vi "Workspace.UI.Update.vi"(8 "error in (no error)":errorcluster, 9 "Data.PendingChange?":bool, 10 "Values":dbl[](array[numeric]), 11 "UI.Refs":T1) -> (0 "error out":errorcluster)   [LabVIEW 2019, in "Diagnostics Workspace Shared.lvlib"]
uses:
  Diagnostics Workspace Shared.lvlib
  Types/UI.Refs.ctl
  Addon/Addon Shared/Types/Command.New.ctl
  SubModules/CAN-Streaming-Support/Source/Addon/Addon Shared/Types/Type Filter.ctl
  Addon/Addon Shared/Diagnostics Addon Shared.lvlib
  SubModules/CAN-Streaming-Support/Source/Addon/Addon Shared/CAN Stream Support Shared.lvlib
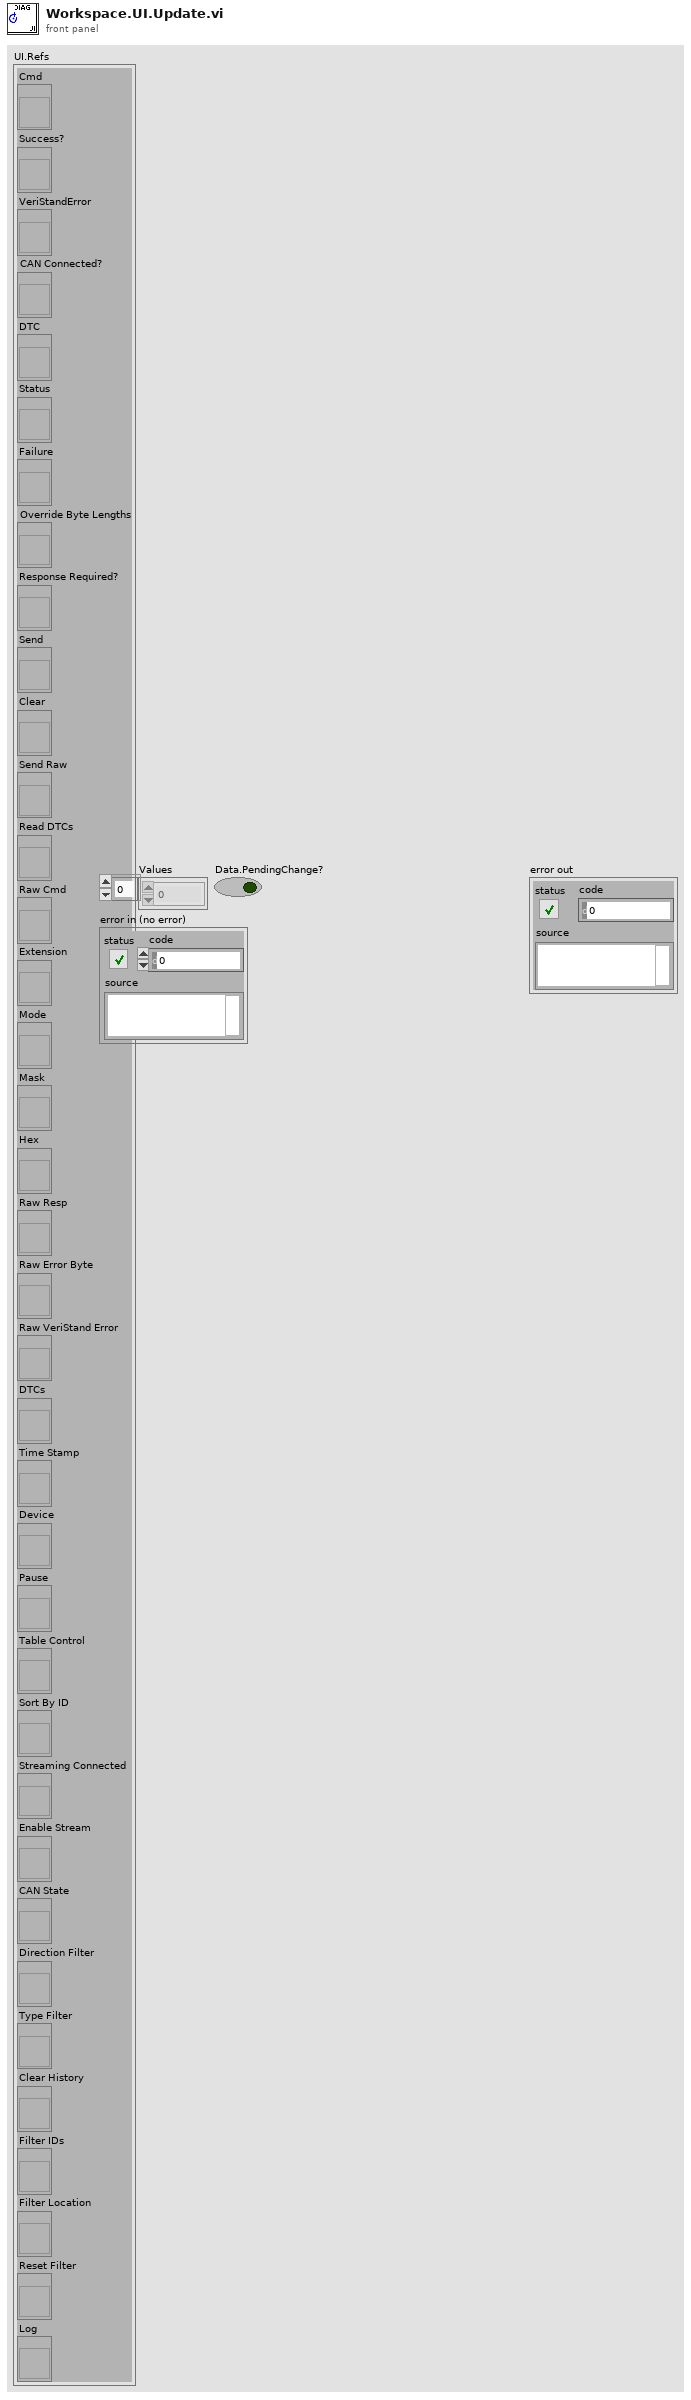
[diagram p1: front panel]
types:
  T1 = typedef "Diagnostics Workspace Shared.lvlib/UI.Refs.ctl" = cluster{"Cmd":refnum<vi>, "Success?":refnum<vi>, "VeriStandError":refnum<vi>, "CAN Connected?":refnum<vi>, "DTC":refnum<vi>, "Status":refnum<vi>, "Failure":refnum<vi>, "Override Byte Lengths":refnum<vi>, "Response Required?":refnum<vi>, "Send":refnum<vi>, "Clear":refnum<vi>, "Send Raw":refnum<vi>, "Read DTCs":refnum<vi>, "Raw Cmd":refnum<vi>, "Extension":refnum<vi>, "Mode":refnum<vi>, "Mask":refnum<vi>, "Hex":refnum<vi>, "Raw Resp":refnum<vi>, "Raw Error Byte":refnum<vi>, "Raw VeriStand Error":refnum<vi>, "DTCs":refnum<vi>, "Time Stamp":refnum<vi>, "Device":refnum<vi>, "Pause":refnum<vi>, "Table Control":refnum<vi>, "Sort By ID":refnum<vi>, "Streaming Connected":refnum<vi>, "Enable Stream":refnum<vi>, "CAN State":refnum<vi>, "Direction Filter":refnum<vi>, "Type Filter":refnum<vi>, "Clear History":refnum<vi>, "Filter IDs":refnum<vi>, "Filter Location":refnum<vi>, "Reset Filter":refnum<vi>, "Log":refnum<vi>}
  T2 = typedef "Command.New.ctl" = enum8{"None", "Clear Status Channels", "Read All DIDs", "Read All PIDs", "Configure and Start DPIDs", "Stop DPIDs"}
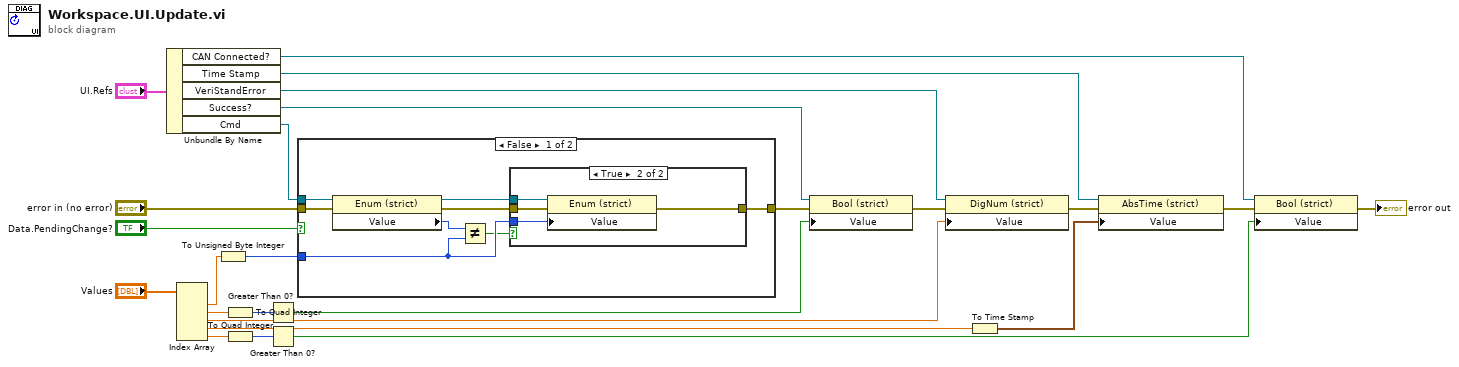
[diagram p0: block diagram]
diagram:
  n1 = Unbundle By Name("UI.Refs") -> ("CAN Connected?"=w10:refnum<vi>, "Time Stamp"=w13:refnum<vi>, "VeriStandError"=w14:refnum<vi>, "Success?"=w15:refnum<vi>, "Cmd"=w6:refnum<vi>)
  n2 = Index Array(array="Values") -> (element #1=w22:dbl, element #2=w7:dbl, element #3=w3:dbl, element #4=w2:dbl, element #5=w1:dbl)  [unwired: 5 in]
  n3 = To Unsigned Byte Integer(number=w22) -> (unsigned 8bit integer=w18:u8)
  n4 = To Quad Integer(1:w7) -> (0:w20:i64)
  n5 = To Quad Integer(1:w1) -> (0:w9:i64)
  n6 = Greater Than 0?(x=w20) -> (x > 0?=w21:bool)
  n7 = Greater Than 0?(x=w9) -> (x > 0?=w8:bool)
  n8 = case shown="False" "Data.PendingChange?" {
    tunnel: [w26 w39] -> w24
    tunnel: "error in (no error)" -> [w33 w39]
    tunnel: w6 -> [w28 _]
    tunnel: w18 -> [w30 _]
    frame False {
      n9 = property class="Enum (strict)"(reference=w28, error in=w33) -> (reference out=w27:refnum<vi>, error out=w32:errorcluster, "Value"=w31:T2)
      n10 = Not Equal?(x=w31, y=w30) -> (x != y?=w29:bool)
      n11 = case shown="True" w29 {
        tunnel: [w34 w35] -> w26
        tunnel: w32 -> [w34 w38]
        tunnel: w27 -> [_ w37]
        tunnel: w30 -> [_ w36]
        frame False {
        }
        frame True {
          n12 = property class="Enum (strict)"(reference=w37, error in=w38, "Value"=w36) -> (error out=w35:errorcluster)  [unwired: 1 out]
        }
      }
    }
    frame True {
    }
  }
  n13 = property class="Bool (strict)"(reference=w15, error in=w24, "Value"=w21) -> (error out=w4:errorcluster)  [unwired: 1 out]
  n14 = property class="DigNum (strict)"(reference=w14, error in=w4, "Value"=w3) -> (error out=w25:errorcluster)  [unwired: 1 out]
  n15 = To Time Stamp(1:w2) -> (0:w5:timestamp)
  n16 = property class="AbsTime (strict)"(reference=w13, error in=w25, "Value"=w5) -> (error out=w12:errorcluster)  [unwired: 1 out]
  n17 = property class="Bool (strict)"(reference=w10, error in=w12, "Value"=w8) -> (error out=→"error out":errorcluster)  [unwired: 1 out]
